vi "GT Get Capture Width.vi"(7 "count":i16, 8 "error in (no error)":errorcluster caption="错误输入（无错误）", 9 "pWidth":i16, 10 "trigger":i16, 11 "cardNum":i16) -> (0 "error out":errorcluster caption="错误输出", 1 "pWidth out":i16, 3 "function return":i16)   [LabVIEW 2020, in "gts.lvlib"]
doc: "GT_API GT_GetCaptureWidth(short cardNum,short trigger,short *pWidth,short count=1);"
uses:
  gts.lvlib
  dll/32bit/multi_card/gts.dll
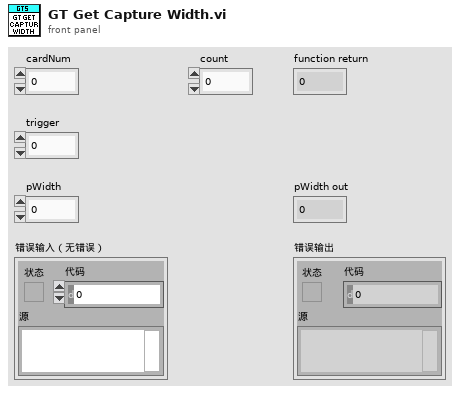
[diagram p1: front panel]
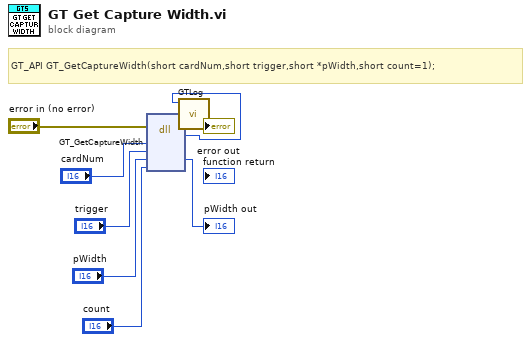
[diagram p0: block diagram]
diagram:
  # "GT_API GT_GetCaptureWidth(short cardNum,short trigger,short *pWidth,short count=1);"
  n1 = dll-call lib="C:/1228/dll/32bit/multi_card/gts.dll" fn="GT_GetCaptureWidth"(error in="error in (no error)", "cardNum"="cardNum", "trigger"="trigger", "pWidth"="pWidth", "count"="count") -> (error out=w3:errorcluster, w1:i16, "pWidth"=→"pWidth out":i16)  [unwired: 5 in, 1 out]
  n2 = call "GTLog.vi"("error in (no error)"=w3, "Numeric"=w1) -> ("error out"=→"error out":errorcluster)  [unwired: 9 in]
